vi "meTEC_Read_ID 1200_Temperature Stability Detection.vi"(6 "Instance (1)":u8=1, 8 "error in (no error)":errorcluster, 9 "TEC Configuration_IN":T1={"VISA resource name"="", "Device Address"=2}, 11 "Sequence No.":u16=5552) -> (0 "error out":errorcluster, 1 "TEC Configuration_OUT":T1={"VISA resource name"="", "Device Address"=2}, 2 "Temperature is Stable? [String] (ID 1200)":string, 3 "Temperature is Stable? [I32)] (ID 1200)":i32)   [LabVIEW 2019]
uses:
  TypeDefs/meTEC_Configuration.ctl
panel:
  # "--- Inputs ---"
  # "--- Outputs ---"
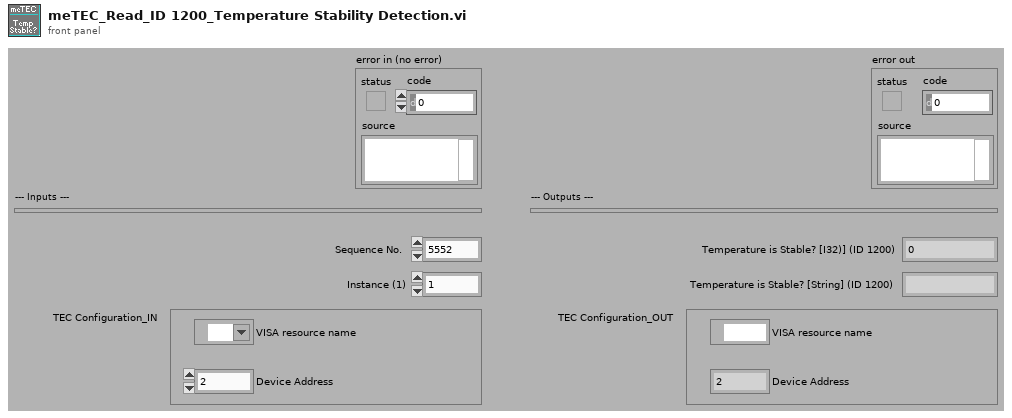
[diagram p1: front panel]
types:
  T1 = typedef "meTEC_Configuration.ctl" = cluster{"VISA resource name":refnum<visa-resource-name>, "Device Address":u16}
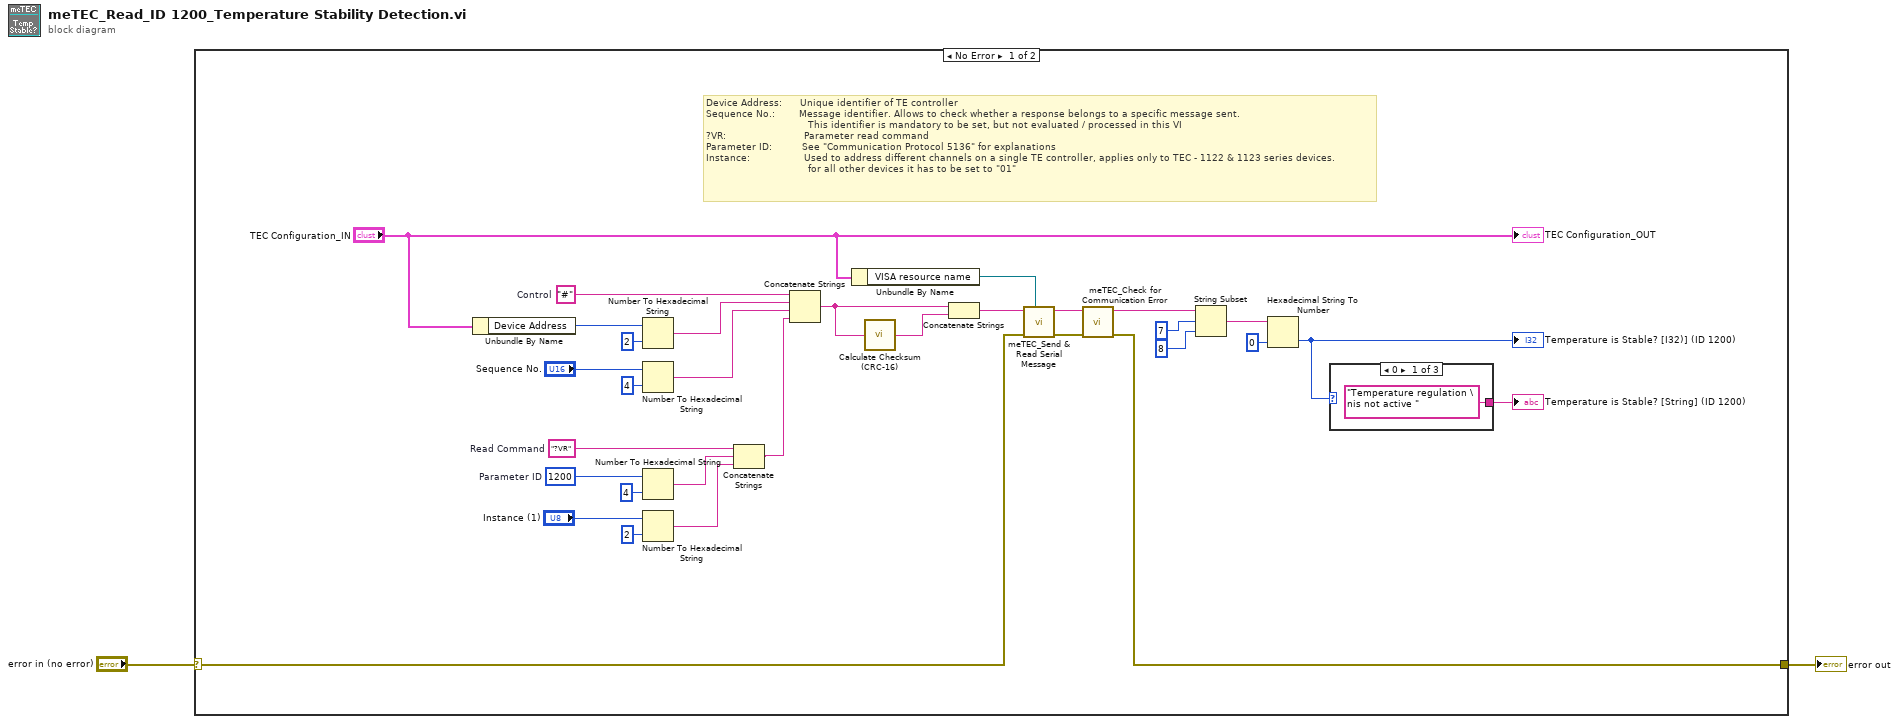
[diagram p0: block diagram]
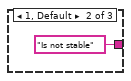
[diagram p2: hidden frame]
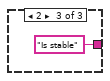
[diagram p3: hidden frame]
diagram:
  n1 = case shown="No Error" "error in (no error)" {
    selector: "error in (no error)" -> [w16 w37]
    tunnel: [w5 w37] -> w2
    frame No Error {
      w22 = 1200  # Parameter ID
      w23 = "?VR"  # Read Command
      w31 = "#"  # Control
      # "Device Address:      Unique identifier of TE controller\nSequence No.:        Message identifier. Allows to check whether a response belongs to a specific message sent.\n                                  This identifier is mandatory to be set, but not evaluated / processed in this VI\n?VR:                          Parameter read command\nParameter ID:          See \"Communication Protocol 5136\" for explanations\nInstance:                  Used to address different channels on a single TE controller, applies only to TEC - 1122 & 1123 series devices.\n                                  for all other devices it has to be set to \"01\""
      n2 = Unbundle By Name("TEC Configuration_IN") -> ("Device Address"=w11:u16)
      n3 = Number To Hexadecimal String(1:i16 2 ("width (-)"), 2:w11) -> (0:w26:string)
      n4 = Number To Hexadecimal String(1:i16 4 ("width (-)"), 2:"Sequence No.") -> (0:w30:string)
      n5 = Number To Hexadecimal String(1:i16 4 ("width (-)"), 2:w22) -> (0:w24:string)
      n6 = Number To Hexadecimal String(1:i16 2 ("width (-)"), 2:"Instance (1)") -> (0:w13:string)
      n7 = Concatenate Strings(w23, w24, w13) -> (w20:string)
      n8 = Concatenate Strings(w31, w26, w30, w20) -> (w29:string)
      n9 = Unbundle By Name("TEC Configuration_IN") -> ("VISA resource name"=w12:refnum<visa-resource-name>)
      n10 = call "Calculate Checksum (CRC-16).vi"("Message"=w29) -> ("CRC [String]"=w28:string)  [unwired: 1 in]
      n11 = Concatenate Strings(w29, w28) -> (w25:string)
      n12 = call "meTEC_Send & Read Serial Message.vi"("VISA resource name"=w12, "error in (no error)"=w16, "Serial Message"=w25) -> ("error out"=w15:errorcluster, "Serial Message_Read"=w4:string)  [unwired: 7 in]
      n13 = call "meTEC_Check for Communication Error.vi"("error in (no error)"=w15, "Serial Message_IN"=w4) -> ("error out"=w5:errorcluster, "Serial Message_OUT"=w3:string)  [unwired: 8 in]
      n14 = String Subset(string=w3, offset (0)=7, length (rest)=8 ("length (rest)")) -> (substring=w17:string)
      n15 = Hexadecimal String To Number(string=w17, default (0uL)=0 ("default (0 U32)")) -> (number=w8:i32)  [unwired: 1 in, 1 out]
      "Temperature is Stable? [I32)] (ID 1200)" <- w8
      n16 = case shown="0" w8 {
        tunnel: ["Temperature regulation \nis not active " "Is not stable" "Is stable"] -> w7
        frame 0 {
        }
        frame 1, Default {
        }
        frame 2 {
        }
      }
      "Temperature is Stable? [String] (ID 1200)" <- w7
      "TEC Configuration_OUT" <- "TEC Configuration_IN"
    }
    frame Error {
    }
  }
  "error out" <- w2
